vi "Get Cont RF.vi"(0 "instrument handle":refnum<k15>, 1 "Skip Frames":i32, 2 "No Reverse":bool, 3 "file name":string, 5 "Num of Frames":i32, 9 "Num of Vectors":i32, 11 "error out":errorcluster, 12 "address":i16) -> (6 "Array out":i8[][](array[numeric]), 8 "Dig Word Size":u16)   [LabVIEW 2022 SP3]
uses:
  Motion Controllers/-MotionRoutines/MotionGlobals.vi
  <instrlib>/vi.lib/Platform/portaccess.llb/Out Port32.vi
  <vilib>/Platform/TimedLoop/XDataNode/XDataNode.xnode
  <vilib>/Platform/TimedLoop/XDataNode/nitl_modes.ctl
  <vilib>/Platform/TimedLoop/XDataNode/XDNodeRunTimeDep.lvlib
  <vilib>/Platform/TimedLoop/XDataNode/wakeup.ctl
  <vilib>/Platform/TimedLoop/XDataNode/timing_clust.ctl
  <instrlib>/niScope/Acquire/Fetch/niScope Multi Fetch Binary 8.vi
  -ScanSystem/DataHandling/ReverseDataI8.vi
  Acqiris/-AcqirisRoutines/VScaleInfoAcq.vi
panel:
  out "frame time":u32
  out "Records Done":i32
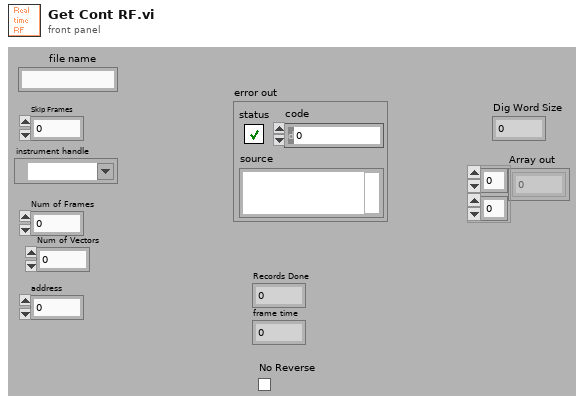
[diagram p1: front panel]
types:
  T1 = typedef "XDNodeRunTimeDep.lvlib/timing_clust.ctl" = cluster{"Expected End [f-1]":u64, "Actual End [f-1]":u64, "Finished Late? [f-1]":bool, "Expected End [i-1]":u64, "Actual End [i-1]":u64, "Finished Late? [i-1]":bool, "Expected Start [i]":u64, "Actual Start [i]":u64, "Expected Start [f]":u64, "Actual Start [f]":u64, "Source Name":string, "Structure Name":string, "Period":i64, "Deadline":i64, "Offset":i64, "Start":i64, "Priority":i32, "Timeout":i32, "Mode":T2, "Wakeup Reason":T3, "Error":errorcluster, "Source Type":string, "Secondary Source Type":string, "Global End Time":u64, "Global Start Time":u64, "Frame Duration":u64, "Iteration Duration":u64, "Assigned CPU":i32, "I/O Scan Engine Mode":u32}
  T2 = typedef "XDNodeRunTimeDep.lvlib/nitl_modes.ctl" = enum32{"No Change", "Process missed periods, maintain original phase", "Discard missed periods, maintain original phase", "Process missed periods, ignore original phase", "Discard missed periods, ignore original phase"}
  T3 = typedef "XDNodeRunTimeDep.lvlib/wakeup.ctl" = enum32{"Normal", "Aborted", "Asynchronous wakeup", "Timing source error", "Timed loop error", "Timeout"}
  T4 = cluster{"actualSamples":i32, "absoluteInitialX":dbl, "relativeInitialX":dbl, "xIncrement":dbl, "offset":dbl, "gain":dbl, "reserved1":dbl, "reserved2":dbl}[]
  T5 = cluster{"actualSamples":i32, "absoluteInitialX":dbl, "relativeInitialX":dbl, "xIncrement":dbl, "offset":dbl, "gain":dbl, "reserved1":dbl, "reserved2":dbl}
  T6 = cluster{sgl, "Gain [dB]  ":sgl, "Atten (dB)":sgl}
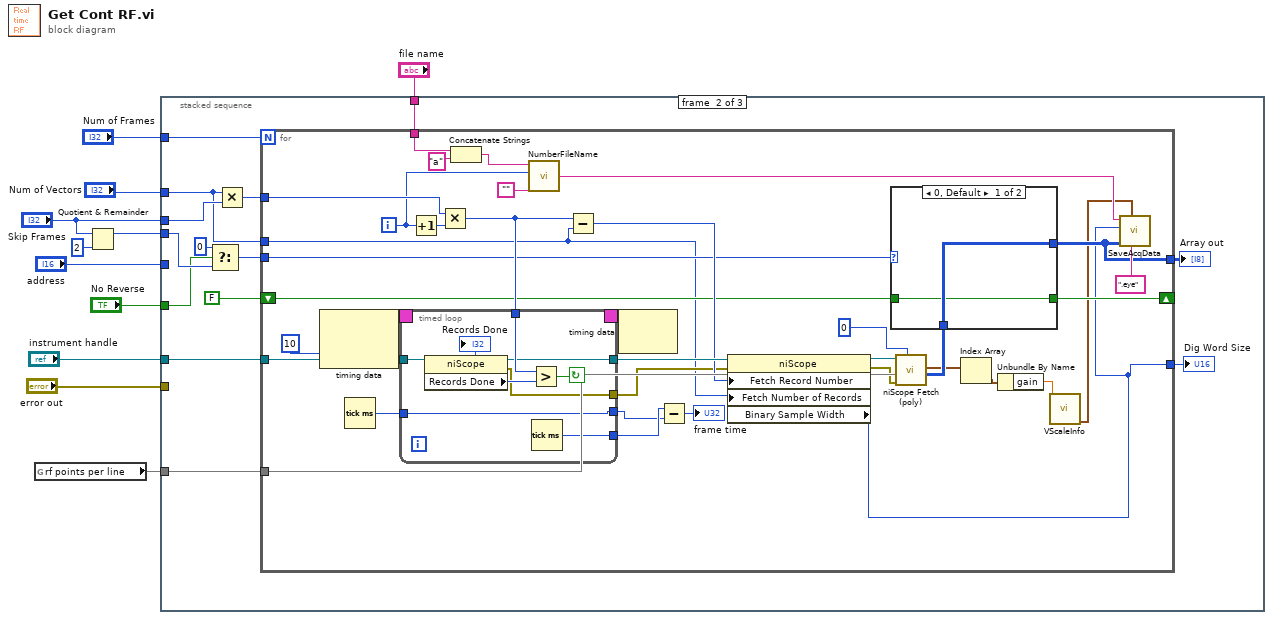
[diagram p0: block diagram]
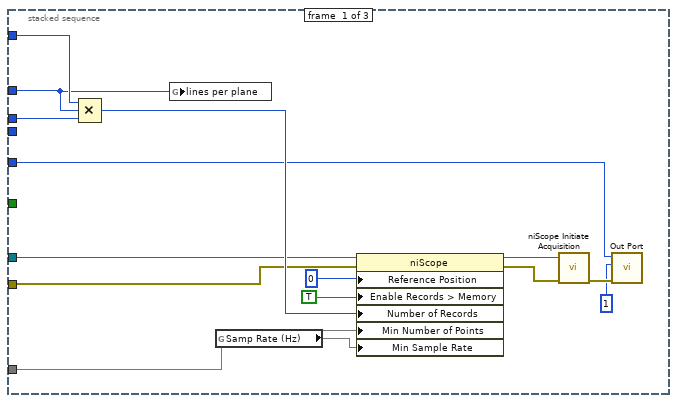
[diagram p2: hidden frame]
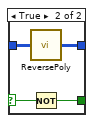
[diagram p4: hidden frame]
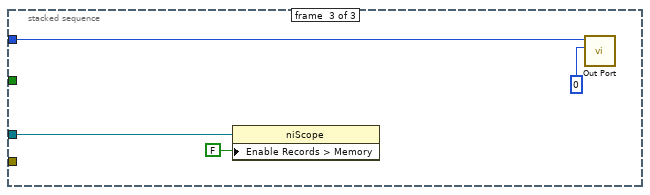
[diagram p5: hidden frame]
diagram:
  n1 = global read "MotionGlobals.vi" "rf points per line"() -> (w6)
  n2 = Quotient & Remainder(x="Skip Frames", y=2) -> (x-y*floor(x/y)=w2:i32)  [unwired: 1 out]
  n3 = stacked-sequence {
    tunnel: "error out" -> [w20 _ _]
    tunnel: "instrument handle" -> [w19 w39 w104]
    tunnel: "address" -> [w18 _ w106]
    tunnel: "Num of Frames" -> [w17 w38 _]
    tunnel: "Num of Vectors" -> [w14 w35 _]
    tunnel: w6 -> [w16 w40 _]
    tunnel: "Skip Frames" -> [w12 w37 _]
    tunnel: "file name" -> [_ w34 _]
    tunnel: w2 -> [_ w32 _]
    tunnel: "No Reverse" -> [_ w30 _]
    frame #0 {
      n4 = Compound Arithmetic op=MULTIPLY(w17, w14, w12) -> (w21:i32)
      n5 = global write "MotionGlobals.vi" "lines per plane"(w14) -> ()
      n6 = global read "MotionGlobals.vi" "Samp Rate (Hz)"() -> (w26)
      n7 = property class="niScope"(reference=w19, error in=w20, "Reference Position"=0, "Enable Records > Memory"=TRUE ("Horizontal:Enable Records > Memory"), "Number of Records"=w21, "Min Number of Points"=w16, "Min Sample Rate"=w26) -> (reference out=w22:refnum<k15>, error out=w13:errorcluster)
      n8 = call <instrlib>:"niScope Initiate Acquisition.vi"("instrument handle"=w22, "error in"=w13) -> ("error out"=w24:errorcluster)  [unwired: 13 out]
      n9 = call-poly <instrlib>:"Out Port.vi"("error in (no error)"=w24, "write value"=1, "address"=w18) -> ()  [unwired: 7 out]
    }
    frame #1 {
      n10 = Select(t=0, s=w30, f=w32) -> (s? t:f=w31:i32)
      n11 = Multiply(x=w35, y=w37) -> (x*y=w36:i32)
      n12 = for {
        N: w38 -> [_]
        tunnel: w40 -> [w76]
        tunnel: w39 -> [w75]
        tunnel: w36 -> [w73]
        tunnel: w35 -> [w47]
        tunnel: w34 -> [w63]
        shift-right: [w57] -> _
        shift-left: FALSE -> [w58]
        tunnel: w31 -> [w56]
        tunnel: [w46] -> w28
        tunnel: [w42] -> w27
        i -> [w65]
        n13 = node-c288(i64 10 ("Period")) -> (w55:T1)  [unwired: 1 out]
        n14 = Tick Count (ms)() -> (millisecond timer value=w52:u32)
        n15 = Increment(x=w65) -> (x+1=w74:i32)
        n16 = Multiply(x=w73, y=w74) -> (x*y=w70:i32)
        n17 = timed-loop {
          tunnel: w75 -> [w84]
          tunnel: w70 -> [w83]
          tunnel: [w81] -> w72
          tunnel: [w79] -> w68
          timing: w55 -> [_]
          timing-out: [_] -> w54
          tunnel: [w78] -> w50
          tunnel: w52 -> [w78]
          tunnel: [w77] -> w51
          stop <- w82 continue-if-true
          n18 = property class="niScope"(reference=w84) -> (reference out=w81:refnum<k15>, error out=w79:errorcluster, "Records Done"=w80:i32)  [unwired: 1 in]
          "Records Done" <- w80
          n19 = Greater?(x=w83, y=w80) -> (0:w82:bool)
          n20 = Tick Count (ms)() -> (millisecond timer value=w77:u32)
        }
        n21 = Concatenate Strings(w63, "a") -> (w62:string)
        n22 = call "NumberFileName.vi"("String"="", "File number"=w65, "file name"=w62) -> ("Numbered File"=w59:string)  [unwired: 1 in]
        n23 = Subtract(x=w70, y=w47) -> (x-y=w69:i32)
        n24 = node-c288(w54) -> ()  [unwired: 1 out]
        n25 = Subtract(x=w51, y=w50) -> (x-y=→"frame time":u32)
        n26 = property class="niScope"(reference=w72, error in=w68, "Fetch Record Number"=w69, "Fetch Number of Records"=w47) -> (reference out=w71:refnum<k15>, error out=w67:errorcluster, "Binary Sample Width"=w42:i32)
        n27 = call-poly <instrlib>:"niScope Fetch (poly).vi"("timeout"=0, "error in"=w67, "numSamples"=w76, "instrument handle"=w71) -> ("wfm"=w60:i8[][], "wfm info"=w45:T4)  [unwired: 1 in, 5 out]
        n28 = case shown="0, Default" w56 {
          tunnel: [w92 w96] -> w46
          tunnel: w60 -> [w92 w95]
          tunnel: w58 -> [w91 w94]
          tunnel: [w91 w93] -> w57
          frame 0, Default {
          }
          frame 1 {
            n29 = case shown="False" w94 {
              selector: w94 -> [w97 w102]
              tunnel: [w98 w99] -> w96
              tunnel: w95 -> [w98 w100]
              tunnel: [w97 w101] -> w93
              frame False {
              }
              frame True {
                n30 = call-poly "ReversePoly.vi"("Array in"=w100) -> ("Array out"=w99:i8[][])
                n31 = Not(x=w102) -> (.not. x?=w101:bool)
              }
            }
          }
        }
        n32 = Index Array(array=w45) -> (element=w44:T5)  [unwired: 1 in]
        n33 = Unbundle By Name(w44) -> ("gain"=w43:dbl)
        n34 = call-poly "VScaleInfo.vi"("vGain scalar"=w43) -> ("Voltage Scale"=w41:T6)  [unwired: 7 in, 2 out]
        n35 = call "SaveAcqData.vi"("Ext"=".eye", "Votage scaling"=w41, "Array"=w46, "Dig Word Size"=w42, "File Name"=w59) -> ()  [unwired: 2 in]
      }
      "Array out" <- w28
      "Dig Word Size" <- w27
    }
    frame #2 {
      n36 = property class="niScope"(reference=w104, "Enable Records > Memory"=FALSE ("Horizontal:Enable Records > Memory")) -> ()  [unwired: 1 in, 2 out]
      n37 = call-poly <instrlib>:"Out Port.vi"("write value"=0, "address"=w106) -> ()  [unwired: 1 in, 7 out]
    }
  }
